vi "duty-cycle-oscillator.vi"(8 "Input State":bool, 9 "time low mS":dbl, 10 "time high mS":dbl, 11 "lastEvent mS":u32) -> (0 "output state":bool, 1 "lastState":bool, 2 "Countdown Timer (mS)":u32, 3 "lastEvent ms Out":u32)   [LabVIEW 2020]
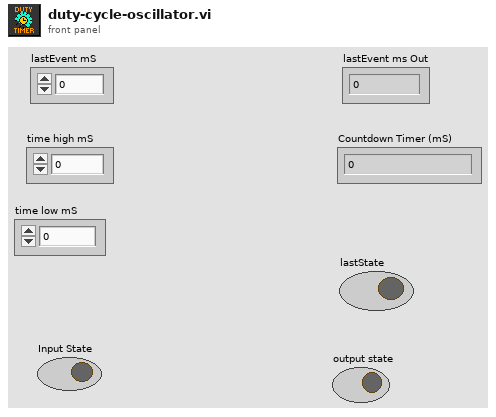
[diagram p1: front panel]
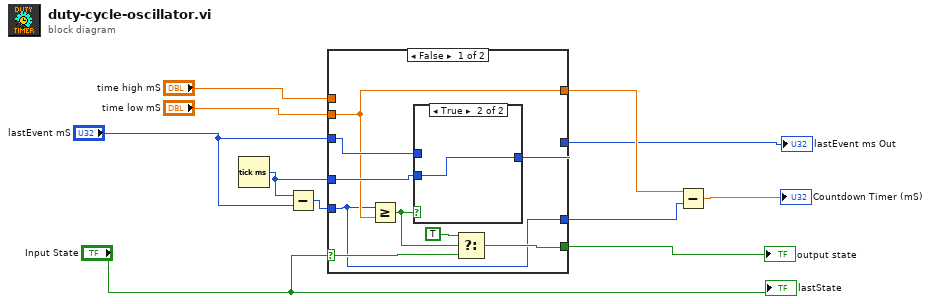
[diagram p0: block diagram]
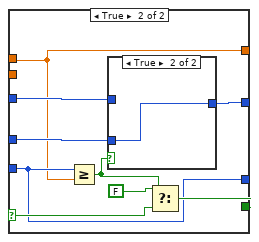
[diagram p3: hidden frame]
diagram:
  n1 = Tick Count (ms)() -> (millisecond timer value=w1:u32)
  n2 = Subtract(x=w1, y="lastEvent mS") -> (x-y=w9:u32)
  n3 = case shown="False" "Input State" {
    selector: "Input State" -> [w17 w27]
    tunnel: w9 -> [w12 w24]
    tunnel: "time high mS" -> [_ w23]
    tunnel: w1 -> [w20 w31]
    tunnel: "lastEvent mS" -> [w19 w30]
    tunnel: [w18 w29] -> w3
    tunnel: "time low mS" -> [w13 _]
    tunnel: [w14 w28] -> w7
    tunnel: [w12 w24] -> w10
    tunnel: [w13 w23] -> w11
    frame False {
      n4 = Greater Or Equal?(x=w12, y=w13) -> (x >= y?=w16:bool)
      n5 = case shown="True" w16 {
        tunnel: w20 -> [_ w22]
        tunnel: w19 -> [w21 _]
        tunnel: [w21 w22] -> w18
        frame False {
        }
        frame True {
        }
      }
      n6 = Select(t=TRUE, s=w16, f=w17) -> (s? t:f=w14:bool)
    }
    frame True {
      n7 = Greater Or Equal?(x=w24, y=w23) -> (x >= y?=w26:bool)
      n8 = case shown="True" w26 {
        tunnel: w31 -> [_ w33]
        tunnel: w30 -> [w32 _]
        tunnel: [w32 w33] -> w29
        frame False {
        }
        frame True {
        }
      }
      n9 = Select(t=FALSE, s=w26, f=w27) -> (s? t:f=w28:bool)
    }
  }
  "output state" <- w7
  "lastEvent ms Out" <- w3
  n10 = Subtract(x=w11, y=w10) -> (x-y=→"Countdown Timer (mS)":dbl)
  "lastState" <- "Input State"
